vi "Tree(SubVI).vi"() -> ()   [LabVIEW 2013]
uses:
  FYP_LabviewGlobal(SubVI).vi
  <vilib>/addons/database/Connection.llb/DB Tools Open Connec (String).vi
  <vilib>/addons/database/_DB Variant To Data/Database Variant To Data.xnode
  <vilib>/addons/database/NI_Database_API.lvlib
panel:
  out "Time Stamp":timestamp format="%<%I:%M:%S %p\n%x>T"
  out "Active Cell:String":string
  out "Get Theme":string
  out "Get Topic":string
  out "Get Paper":string
  in  "LogOut":bool
  out "AdminNo":string
  out "Name":string
  in  "Tree 4":string(tree)
  # "Admin No:"
  # "Name:"
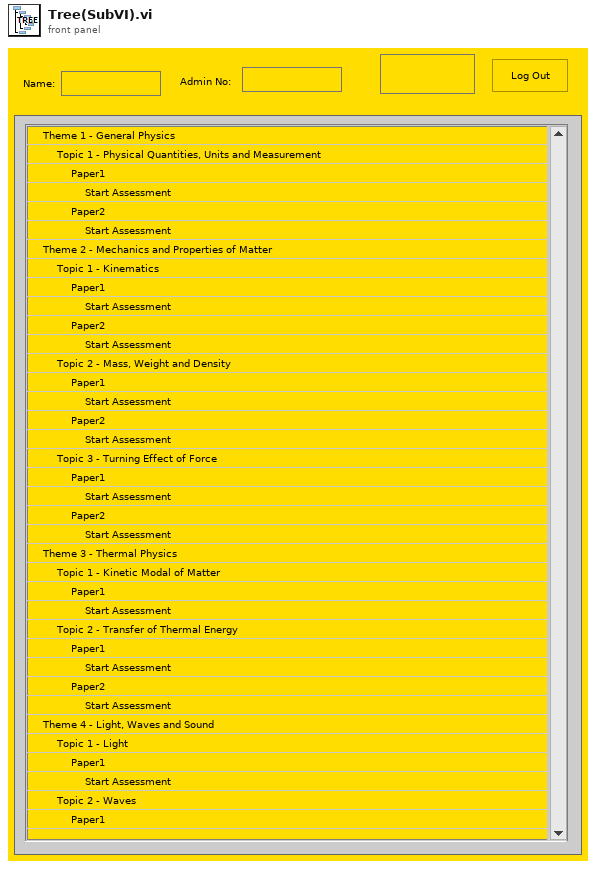
[diagram p1: front panel]
types:
  T1 = typedef "NI_Database_API.lvlib/Conn ObjectReference.ctl" = refnum<k1>
  T2 = cluster{"AdminNo":string, "Get Login Time":string, "date/time string":string}
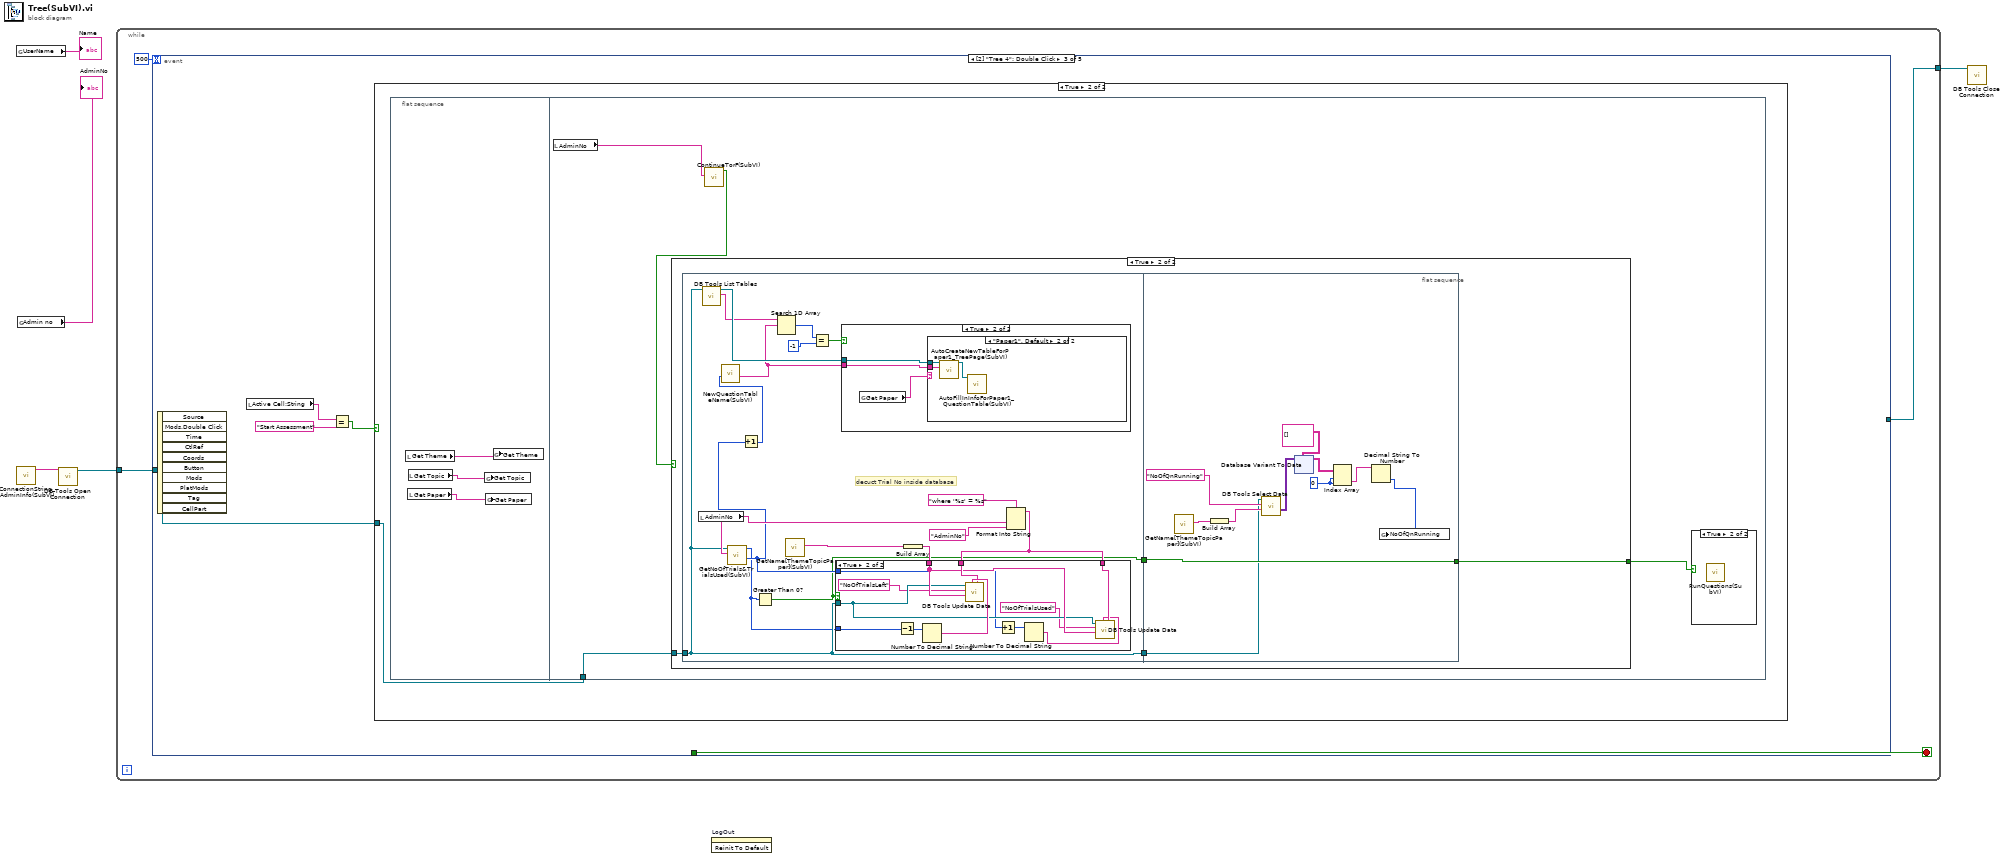
[diagram p0: block diagram]
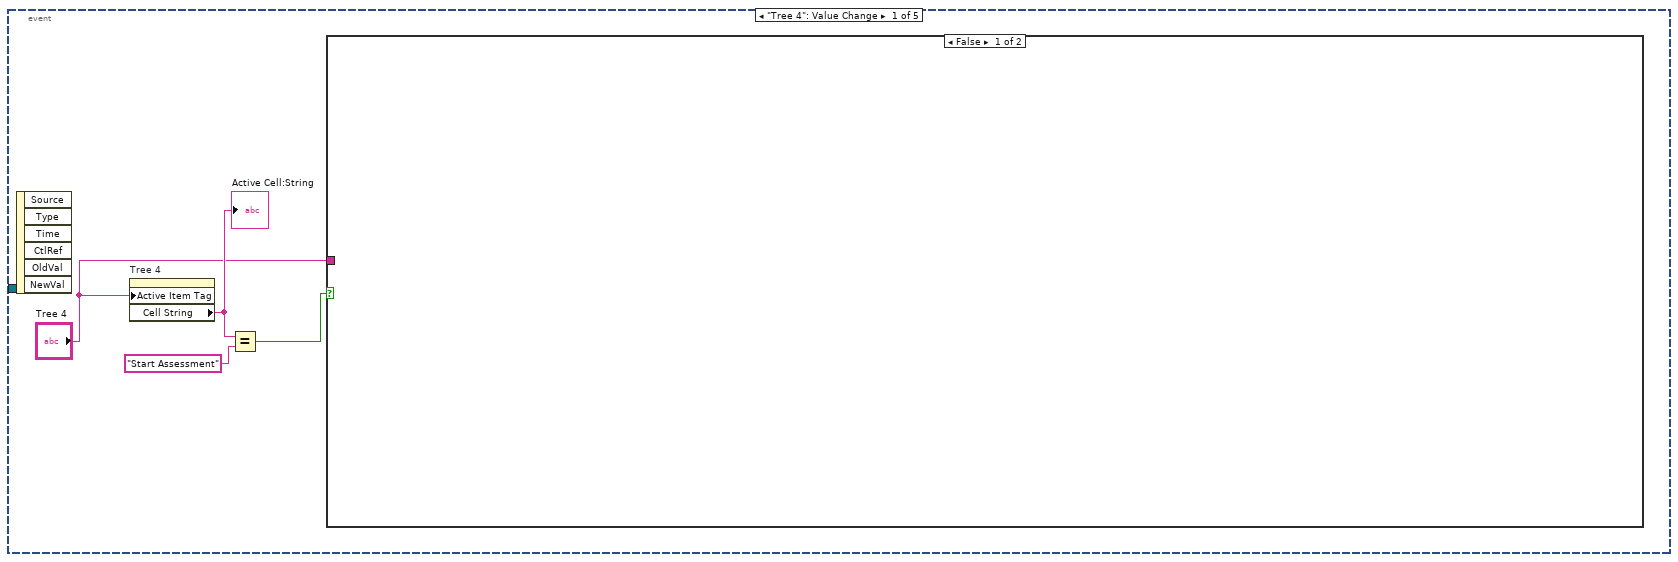
[diagram p2: hidden frame]
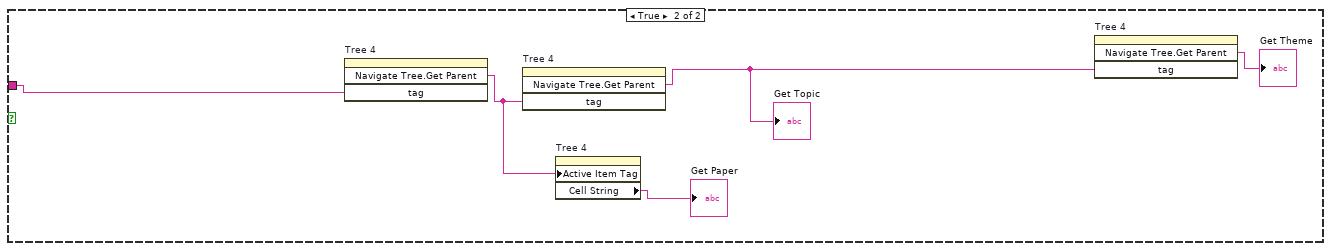
[diagram p3: hidden frame]
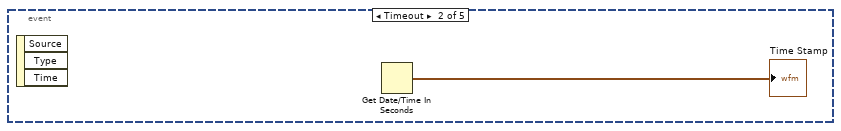
[diagram p4: hidden frame]
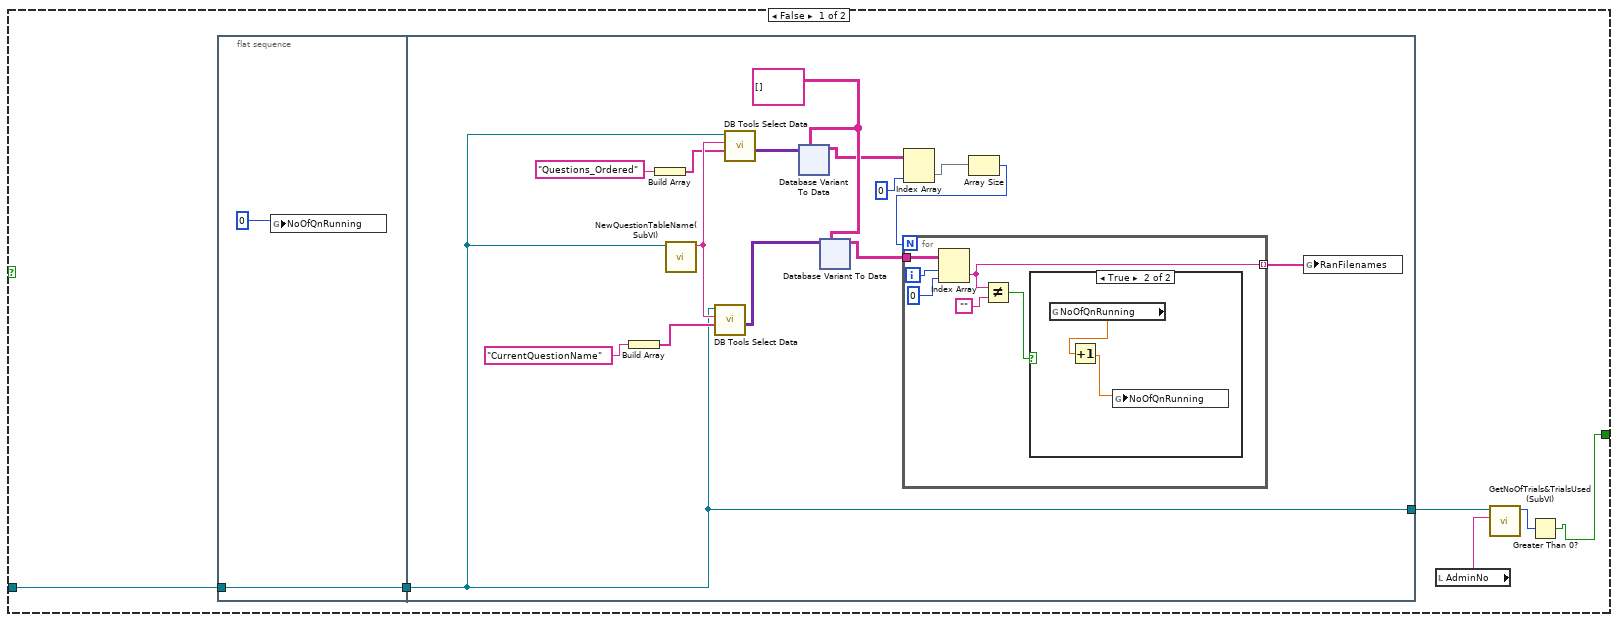
[diagram p6: hidden frame]
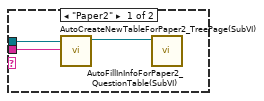
[diagram p9: hidden frame]
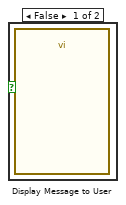
[diagram p11: hidden frame]
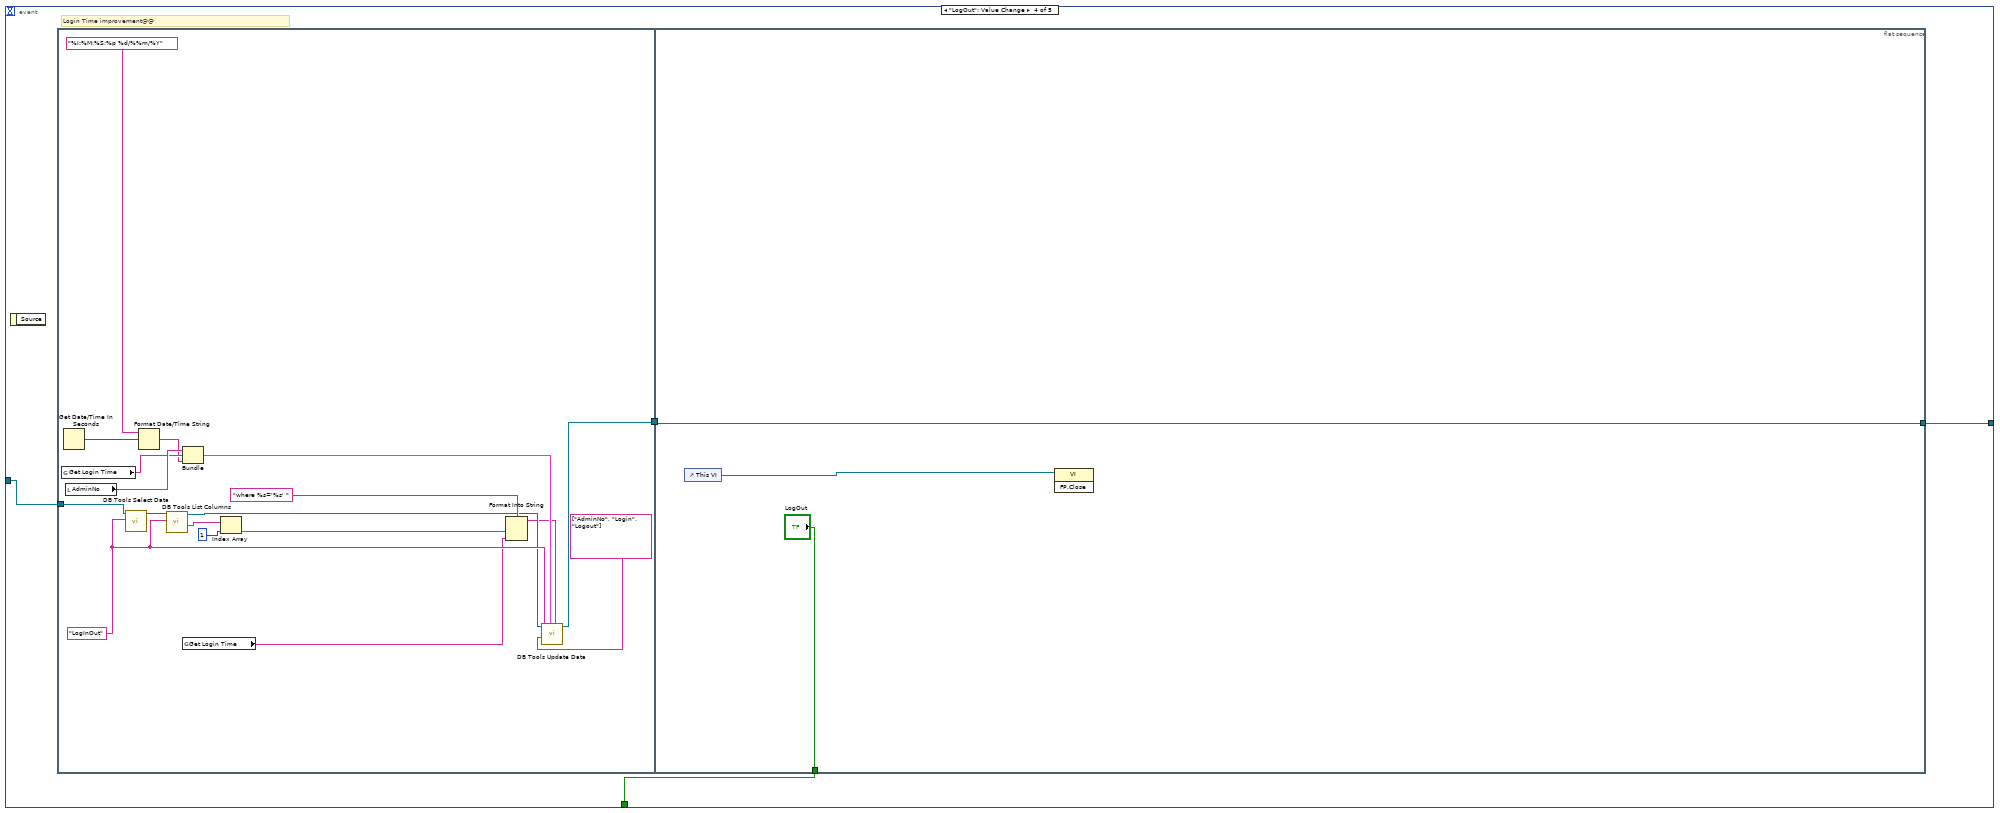
[diagram p12: hidden frame]
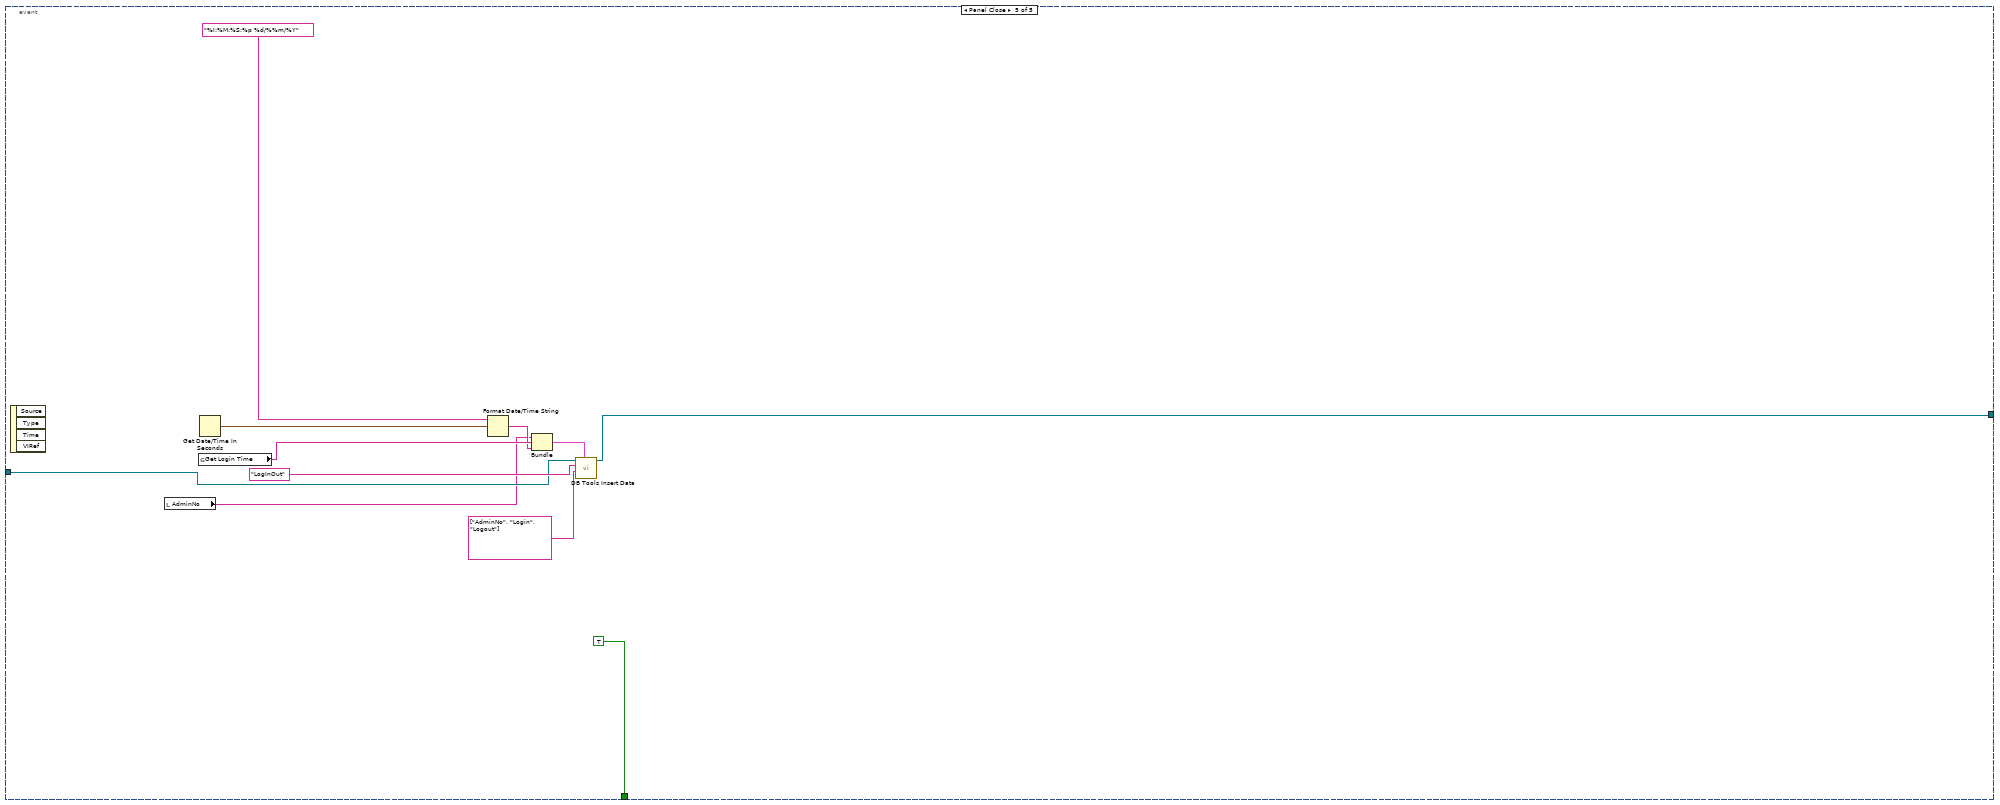
[diagram p13: hidden frame]
diagram:
  n1 = global read "FYP_LabviewGlobal(SubVI).vi" "UserName"() -> (→"Name":string)
  n2 = call "ConnectionString_AdminInfo(SubVI).vi"() -> ("ConnectionString"=w3:string)  [unwired: 11 in]
  n3 = global read "FYP_LabviewGlobal(SubVI).vi" "Admin no"() -> (→"AdminNo":string)
  n4 = call-poly <vilib>:"DB Tools Open Connection.vi"("connection information"=w3) -> ("connection reference"=w2:T1)  [unwired: 7 in, 1 out]
  n5 = while {
    tunnel: w2 -> [w8]
    tunnel: [w7] -> w1
    stop <- w6 stop-if-true
    n6 = event shown="[2] \"Tree 4\": Double Click" {
      selector: _ -> [_ _ _ _ _]
      dyn-events: _ -> [_ _ _ _ _]
      timeout: 500 -> [_ _ _ _ _]
      tunnel: w8 -> [_ _ w20 w251 w276]
      tunnel: [_ _ _ w250 w274] -> w7
      tunnel: [_ _ _ w248 TRUE] -> w6
      event "Tree 4": Value Change {
        n7 = event-data() -> ()  [unwired: 1 in, 6 out]
        n8 = property on="Tree 4" class="Tree (strict)"("Active Item Tag"="Tree 4") -> ("Cell String"=w12:string)  [unwired: 2 in, 2 out]
        "Active Cell:String" <- w12
        n9 = Equal?(x=w12, y="Start Assessment") -> (x = y?=w11:bool)
        n10 = case shown="False" w11 {
          tunnel: "Tree 4" -> [_ w14]
          frame False {
          }
          frame True {
            n11 = invoke on="Tree 4" class="Tree (strict)" method="Navigate Tree.Get Parent"("tag"=w14) -> ("Navigate Tree:Get Parent"=w18:string)  [unwired: 3 in, 3 out]
            n12 = invoke on="Tree 4" class="Tree (strict)" method="Navigate Tree.Get Parent"("tag"=w18) -> ("Navigate Tree:Get Parent"=w16:string)  [unwired: 3 in, 3 out]
            "Get Topic" <- w16
            n13 = property on="Tree 4" class="Tree (strict)"("Active Item Tag"=w18) -> ("Cell String"=→"Get Paper":string)  [unwired: 2 in, 2 out]
            n14 = invoke on="Tree 4" class="Tree (strict)" method="Navigate Tree.Get Parent"("tag"=w16) -> ("Navigate Tree:Get Parent"=→"Get Theme":string)  [unwired: 3 in, 3 out]
          }
        }
      }
      event Timeout {
        n15 = event-data() -> ()  [unwired: 1 in, 3 out]
        n16 = Get Date/Time In Seconds() -> (seconds since 1Jan1904=→"Time Stamp":timestamp)
      }
      event "Tree 4": Double Click {
        n17 = event-data() -> ()  [unwired: 1 in, 10 out]
        n18 = local read "Active Cell:String"() -> (w23:string)
        n19 = Equal?(x=w23, y="Start Assessment") -> (x = y?=w21:bool)
        n20 = case shown="True" w21 {
          tunnel: w20 -> [_ w24]
          frame False {
          }
          frame True {
            n21 = flat-sequence {
              tunnel: w24 -> [w30]
              frame #0 {
                n22 = local read "Get Theme"() -> (w27:string)
                n23 = local read "Get Paper"() -> (w25:string)
                n24 = local read "Get Topic"() -> (w26:string)
                n25 = global write "FYP_LabviewGlobal(SubVI).vi" "Get Topic"(w26) -> ()
                n26 = global write "FYP_LabviewGlobal(SubVI).vi" "Get Paper"(w25) -> ()
                n27 = global write "FYP_LabviewGlobal(SubVI).vi" "Get Theme"(w27) -> ()
              }
              frame #1 {
                n28 = local read "AdminNo"() -> (w29:string)
                n29 = call "ContinueTorF(SubVI).vi"("AdminNo"=w29) -> ("Boolean"=w28:bool)  [unwired: 10 in]
                n30 = case shown="True" w28 {
                  tunnel: w30 -> [w37 w152]
                  tunnel: [w32 w151] -> w31
                  frame False {
                    n31 = flat-sequence {
                      tunnel: w37 -> [w39]
                      tunnel: [w39] -> w36
                      tunnel: w36 -> [w41]
                      tunnel: [w41] -> w35
                      frame #0 {
                        n32 = global write "FYP_LabviewGlobal(SubVI).vi" "NoOfQnRunning"(0) -> ()
                      }
                      frame #1 {
                        w47 = string[][] []
                        n33 = Build Array("CurrentQuestionName") -> (w54:string[])
                        n34 = Build Array("Questions_Ordered") -> (w48:string[])
                        n35 = call "NewQuestionTableName(SubVI).vi"("connection reference"=w41) -> ("String"=w50:string)  [unwired: 9 in, 1 out]
                        n36 = call <vilib>:"DB Tools Select Data.vi"("columns"=w54, "table"=w50, "connection reference"=w41) -> ("data"=w53:variant[][])  [unwired: 3 in, 2 out]
                        n37 = call <vilib>:"DB Tools Select Data.vi"("columns"=w48, "table"=w50, "connection reference"=w41) -> ("data"=w46:variant[][])  [unwired: 3 in, 2 out]
                        n38 = xnode "Database Variant To Data"("database variant"=w46, "type"=w47) -> ("data"=w45:string[][])  [unwired: 1 in, 1 out]
                        n39 = xnode "Database Variant To Data"("database variant"=w53, "type"=w47) -> ("data"=w51:string[][])  [unwired: 1 in, 1 out]
                        n40 = Index Array(array=w45, index (col)=0 ("disabled index (col)")) -> (element=w43:string[])  [unwired: 1 in]
                        n41 = Array Size(array=w43) -> (size(s)=w42:i32)
                        n42 = for {
                          N: w42 -> [_]
                          tunnel: w51 -> [w104]
                          tunnel: [w99] -> w40 mode=indexing
                          i -> [w103]
                          n43 = Index Array(array=w104, index (row)=w103, index (col)=0 ("disabled index (col)")) -> (element=w99:string)
                          n44 = Not Equal?(x=w99, y="") -> (x != y?=w101:bool)
                          n45 = case shown="True" w101 {
                            frame False {
                            }
                            frame True {
                              n46 = global read "FYP_LabviewGlobal(SubVI).vi" "NoOfQnRunning"() -> (w106:dbl)
                              n47 = Increment(x=w106) -> (x+1=w105:dbl)
                              n48 = global write "FYP_LabviewGlobal(SubVI).vi" "NoOfQnRunning"(w105) -> ()
                            }
                          }
                        }
                        n49 = global write "FYP_LabviewGlobal(SubVI).vi" "RanFilenames"(w40) -> ()
                      }
                    }
                    n50 = local read "AdminNo"() -> (w34:string)
                    n51 = call "GetNoOfTrials&TrialsUsed(SubVI).vi"("Admin no"=w34, "Refnum in"=w35) -> ("NoOfTrials"=w33:i32)  [unwired: 8 in, 1 out]
                    n52 = Greater Than 0?(x=w33) -> (x > 0?=w32:bool)
                  }
                  frame True {
                    n53 = flat-sequence {
                      tunnel: w152 -> [w157]
                      tunnel: [w156] -> w154
                      tunnel: [w157] -> w153
                      tunnel: w154 -> [w194]
                      tunnel: [w194] -> w151
                      tunnel: w153 -> [w193]
                      frame #0 {
                        # "decuct Trial No inside database"
                        n54 = local read "AdminNo"() -> (w162:string)
                        n55 = call <vilib>:"DB Tools List Tables.vi"("connection reference"=w157) -> ("tables"=w166:string[], "connection reference out"=w167:T1)  [unwired: 4 in, 1 out]
                        n56 = call "GetNoOfTrials&TrialsUsed(SubVI).vi"("Admin no"=w162, "Refnum in"=w157) -> ("NoOfTrialsUsed"=w159:i32, "NoOfTrials"=w155:i32)  [unwired: 8 in]
                        n57 = Increment(x=w159) -> (x+1=w158:i32)
                        n58 = call "NewQuestionTableName(SubVI).vi"("For Tree Control"=w158) -> ("For Tree Control"=w160:string)  [unwired: 9 in, 1 out]
                        n59 = Greater Than 0?(x=w155) -> (x > 0?=w156:bool)
                        n60 = Search 1D Array(1D array=w166, element=w160) -> (index of element=w165:i32)  [unwired: 1 in]
                        n61 = call "GetName[ThemeTopicPaper](SubVI).vi"() -> ("Path for Score Table"=w171:string)  [unwired: 11 in]
                        n62 = Equal?(x=w165, y=-1) -> (x = y?=w163:bool)
                        n63 = case shown="True" w163 {
                          tunnel: w167 -> [_ w174]
                          tunnel: w160 -> [_ w173]
                          frame False {
                          }
                          frame True {
                            n64 = global read "FYP_LabviewGlobal(SubVI).vi" "Get Paper"() -> (w172:string)
                            n65 = case shown="\"Paper1\", Default" w172 {
                              tunnel: w174 -> [w177 w180]
                              tunnel: w173 -> [w176 w179]
                              frame "Paper2" {
                                n66 = call "AutoCreateNewTableForPaper2_TreePage(SubVI).vi"("NameOfTable"=w176, "connection reference"=w177) -> ("Refnum out"=w175:T1)  [unwired: 9 in]
                                n67 = call "AutoFillInInfoForPaper2_QuestionTable(SubVI).vi"("Refnum in"=w175) -> ()  [unwired: 11 in]
                              }
                              frame "Paper1", Default {
                                n68 = call "AutoCreateNewTableForPaper1_TreePage(SubVI).vi"("NameOfTable"=w179, "connection reference"=w180) -> ("Refnum out"=w178:T1)  [unwired: 9 in]
                                n69 = call "AutoFillInInfoForPaper1_QuestionTable(SubVI).vi"("Refnum in"=w178) -> ()  [unwired: 11 in]
                              }
                            }
                          }
                        }
                        n70 = Build Array(w171) -> (w170:string[])
                        n71 = Format Into String(format string="where '%s' = %s", w162, "AdminNo") -> (resulting string=w161:string)  [unwired: 2 in, 1 out]
                        n72 = case shown="True" w156 {
                          tunnel: w157 -> [_ w185]
                          tunnel: w170 -> [_ w186]
                          tunnel: w161 -> [_ w191]
                          tunnel: w155 -> [_ w189]
                          tunnel: w161 -> [_ w188]
                          tunnel: w159 -> [_ w184]
                          frame False {
                          }
                          frame True {
                            n73 = Decrement(x=w189) -> (x-1=w190:i32)
                            n74 = Number To Decimal String(number=w190) -> (decimal integer string=w192:string)  [unwired: 1 in]
                            n75 = call <vilib>:"DB Tools Update Data.vi"("condition"=w191, "data"=w192, "columns"=w186, "table"="NoOfTrialsLeft", "connection reference"=w185) -> ()  [unwired: 5 in, 2 out]
                            n76 = Increment(x=w184) -> (x+1=w183:i32)
                            n77 = Number To Decimal String(number=w183) -> (decimal integer string=w187:string)  [unwired: 1 in]
                            n78 = call <vilib>:"DB Tools Update Data.vi"("condition"=w188, "data"=w187, "columns"=w186, "table"="NoOfTrialsUsed", "connection reference"=w185) -> ()  [unwired: 5 in, 2 out]
                          }
                        }
                      }
                      frame #1 {
                        w198 = 0 ("disabled index (col)")
                        n79 = call "GetName[ThemeTopicPaper](SubVI).vi"() -> ("Path for Score Table"=w201:string)  [unwired: 11 in]
                        n80 = Build Array(w201) -> (w202:string[])
                        n81 = call <vilib>:"DB Tools Select Data.vi"("columns"=w202, "table"="NoOfQnRunning", "connection reference"=w193) -> ("data"=w196:variant[][])  [unwired: 3 in, 2 out]
                        n82 = xnode "Database Variant To Data"("database variant"=w196, "type"=string[][] []) -> ("data"=w199:string[][])  [unwired: 1 in, 1 out]
                        n83 = Index Array(array=w199, index (row)=w198, index (col)=w198) -> (element=w197:string)
                        n84 = Decimal String To Number(string=w197) -> (number=w195:i32)  [unwired: 2 in, 1 out]
                        n85 = global write "FYP_LabviewGlobal(SubVI).vi" "NoOfQnRunning"(w195) -> ()
                      }
                    }
                  }
                }
                n86 = case shown="True" w31 {
                  frame False {
                    n87 = call "Display Message to User"() -> ()  [unwired: 10 in, 2 out]
                  }
                  frame True {
                    n88 = call "RunQuestions(SubVI).vi"() -> ()  [unwired: 12 in]
                  }
                }
              }
            }
          }
        }
      }
      event "LogOut": Value Change {
        # "Login Time improvement@@"
        n89 = event-data() -> ()  [unwired: 1 in, 1 out]
        n90 = flat-sequence {
          tunnel: w251 -> [w264]
          tunnel: [w258] -> w249
          tunnel: [w272] -> w250
          tunnel: w249 -> [w272]
          tunnel: ["LogOut"] -> w248
          frame #0 {
            w260 = "LogInOut"
            n91 = global read "FYP_LabviewGlobal(SubVI).vi" "Get Login Time"() -> (w266:string)
            n92 = Get Date/Time In Seconds() -> (seconds since 1Jan1904=w269:timestamp)
            n93 = local read "AdminNo"() -> (w267:string)
            n94 = call <vilib>:"DB Tools Select Data.vi"("table"=w260, "connection reference"=w264) -> ("connection reference out"=w263:T1)  [unwired: 4 in, 2 out]
            n95 = Format Date/Time String(time format string (%c)="%I:%M:%S:%p %d/%%m/%Y", seconds (now)=w269) -> (date/time string=w265:string)  [unwired: 1 in]
            n96 = call <vilib>:"DB Tools List Columns.vi"("table"=w260, "connection reference"=w263) -> ("columns"=w254:string[], "connection reference out"=w259:T1)  [unwired: 2 in, 2 out]
            n97 = Bundle("AdminNo"=w267, "Get Login Time"=w266, "date/time string"=w265) -> (w257:T2)  [unwired: 1 in]
            n98 = global read "FYP_LabviewGlobal(SubVI).vi" "Get Login Time"() -> (w255:string)
            n99 = Index Array(array=w254, index=1 ("disabled index (col)")) -> (element=w253:string)
            n100 = Format Into String(format string="where %s='%s' ", w253, w255) -> (resulting string=w252:string)  [unwired: 2 in, 1 out]
            n101 = call <vilib>:"DB Tools Update Data.vi"("condition"=w252, "data"=w257, "columns"=string[] ["AdminNo", "Login", "Logout"], "table"=w260, "connection reference"=w259) -> ("connection reference out"=w258:T1)  [unwired: 5 in, 1 out]
          }
          frame #1 {
            n102 = control-ref of="This VI"() -> (w270:refnum<vi>)
            n103 = invoke class="VI" method="FP.Close"(reference=w270) -> ()  [unwired: 2 in, 3 out]
          }
        }
      }
      event Panel Close {
        n104 = event-data() -> ()  [unwired: 1 in, 4 out]
        n105 = local read "AdminNo"() -> (w275:string)
        n106 = global read "FYP_LabviewGlobal(SubVI).vi" "Get Login Time"() -> (w281:string)
        n107 = Get Date/Time In Seconds() -> (seconds since 1Jan1904=w283:timestamp)
        n108 = Format Date/Time String(time format string (%c)="%I:%M:%S:%p %d/%%m/%Y", seconds (now)=w283) -> (date/time string=w277:string)  [unwired: 1 in]
        n109 = Bundle("AdminNo"=w275, "Get Login Time"=w281, "date/time string"=w277) -> (w280:T2)  [unwired: 1 in]
        n110 = call <vilib>:"DB Tools Insert Data.vi"("data"=w280, "columns"=string[] ["AdminNo", "Login", "Logout"], "table"="LogInOut", "connection reference"=w276) -> ("connection reference out"=w274:T1)  [unwired: 6 in, 1 out]
      }
    }
  }
  n111 = invoke on="LogOut" class="Bool" method="Reinit To Default"() -> ()  [unwired: 3 in, 3 out]
  n112 = call <vilib>:"DB Tools Close Connection.vi"("connection reference"=w1) -> ()  [unwired: 6 in, 1 out]
